vi "GFITS_LibImgageClose.vi"(8 "error in (no error)":errorcluster, 10 "err in":bool, 11 "fd":u64) -> (0 "error out":errorcluster, 2 "return value":i32)   [LabVIEW 2016]
uses:
  c/lib/libgfits.so
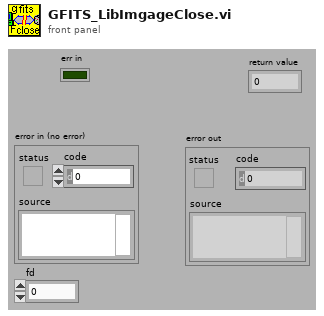
[diagram p1: front panel]
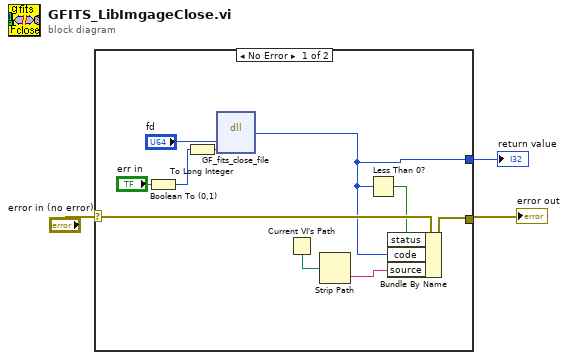
[diagram p0: block diagram]
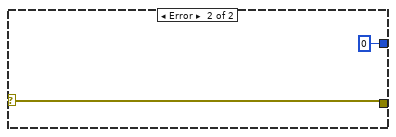
[diagram p2: hidden frame]
diagram:
  n1 = case shown="No Error" "error in (no error)" {
    selector: "error in (no error)" -> [w13 w15]
    tunnel: [w7 0] -> w3
    tunnel: [w9 w15] -> w1
    frame No Error {
      n2 = Boolean To (0,1)(Boolean="err in") -> (0, 1=w5:i16)
      n3 = To Long Integer(number=w5) -> (32bit integer=w4:i32)
      n4 = dll-call lib="home/simager/panview/PAN/Modules/GFITS/private/c/lib/libgfits.so" fn="GF_fits_close_file"("fd"="fd", "err"=w4) -> ("return type"=w7:i32)  [unwired: 5 in, 2 out]
      n5 = Current VI's Path() -> (path=w11:path)
      n6 = Strip Path(path=w11) -> (name=w10:string)  [unwired: 1 out]
      n7 = Less Than 0?(x=w7) -> (x < 0?=w12:bool)
      n8 = Bundle By Name(cluster=w13, "status"=w12, "code"=w7, "source"=w10) -> (w9:errorcluster)
    }
    frame Error {
    }
  }
  "return value" <- w3
  "error out" <- w1
